vi "Control Board - Open.vi"(11 "VISA Refnum in":refnum<visa-resource-name>="COM5") -> (0 "error out":errorcluster, 3 "VISA Refnum out":refnum<visa-resource-name>)   [LabVIEW 2015]
panel:
  out "Boot Message":string
  in  "error in (no error)":errorcluster
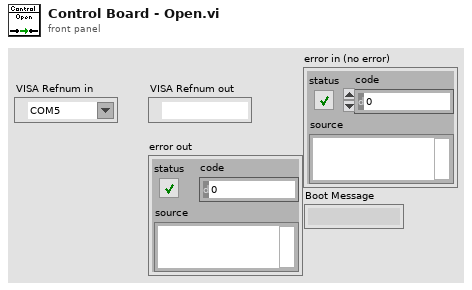
[diagram p1: front panel]
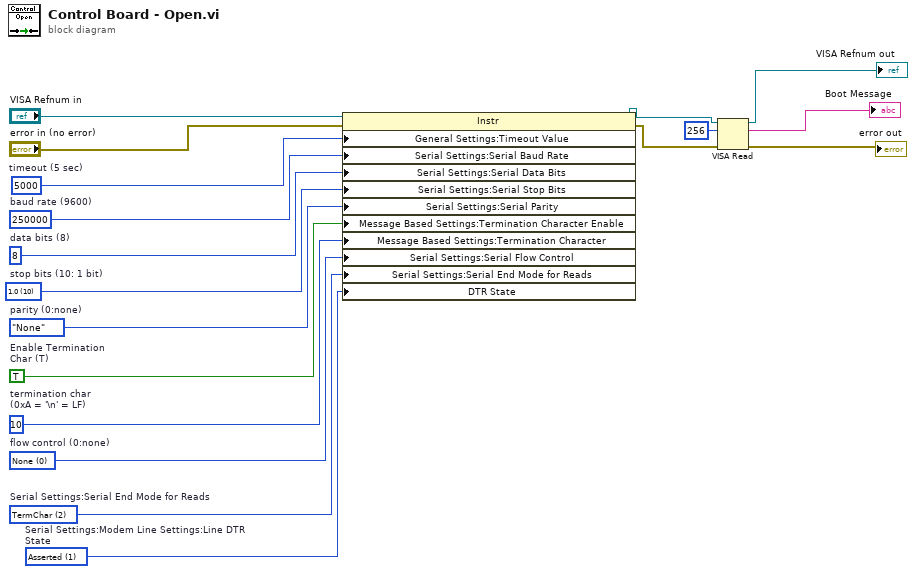
[diagram p0: block diagram]
diagram:
  w18 = i16 1 items=["Unknown"=-1, "Unasserted"=0, "Asserted"=1]  # Serial Settings:Modem Line Settings:Line DTR State
  w9 = u16 8  # data bits (8)
  w13 = u16 2 items=["None", "LastBit", "TermChar"]  # Serial Settings:Serial End Mode for Reads
  w14 = TRUE  # Enable Termination Char (T)
  w15 = u16 0 items=["None", "XON/XOFF", "RTS/CTS", "XON/XOFF & RTS/CTS", "DTR/DSR", "XON/XOFF & DTR/DSR"]  # flow control (0:none)
  w11 = u8 10  # termination char (0xA = '\n' = LF)
  w10 = enum16{"None", "Odd", "Even", "Mark", "Space"}."None"  # parity (0:none)
  w12 = u16 10 items=["1.0"=10, "1.5"=15, "2.0"=20]  # stop bits (10: 1 bit)
  w8 = u32 5000  # timeout (5 sec)
  w17 = u32 250000  # baud rate (9600)
  n1 = property class="Instr"(reference="VISA Refnum in", error in="error in (no error)", "General Settings:Timeout Value"=w8, "Serial Settings:Serial Baud Rate"=w17, "Serial Settings:Serial Data Bits"=w9, "Serial Settings:Serial Stop Bits"=w12, "Serial Settings:Serial Parity"=w10, "Message Based Settings:Termination Character Enable"=w14, "Message Based Settings:Termination Character"=w11, "Serial Settings:Serial Flow Control"=w15, "Serial Settings:Serial End Mode for Reads"=w13, "DTR State"=w18) -> (reference out=w6:refnum<visa-resource-name>, error out=w5:errorcluster)
  n2 = VISA Read(VISA resource name=w6, byte count=u32 256, error in (no error)=w5) -> (VISA resource name out=→"VISA Refnum out":refnum<visa-resource-name>, read buffer=→"Boot Message":string, error out=→"error out":errorcluster)  [unwired: 1 out]
